vi "Example_GUI.vi"() -> ()   [LabVIEW 2016]
panel:
  in  "Device Description":string
  in  "DDS Info":T1
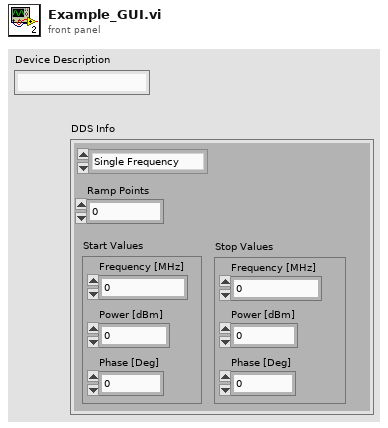
[diagram p1: front panel]
types:
  T1 = cluster{"Start Values":cluster{"Frequency [MHz]":dbl, "Power [dBm]":dbl, "Phase [Deg]":u16}, "Stop Values":cluster{"Frequency [MHz]":dbl, "Power [dBm]":dbl, "Phase [Deg]":u16}, "Ramp Points":i32, "Output Type":enum16{"Single Frequency", "Linear Ramp (dBm)"}}
  T2 = cluster{"Frequency [MHz]":dbl[], "Amplitude (0-1)":dbl[], "Phase":dbl[]}
  T3 = cluster{"Frequency 0 (MHz)":dbl[], "Frequency 1 (MHz)":dbl[], "Amplitude (0-1)":dbl[], "Phase (degrees)":dbl[], "Time (ms)":dbl[], "Sweep Direction (0 = down; 1 = up)":u16[], "Sweeps":bool, "Lock Amp":bool, "Table / Sequence":bool}
  T4 = cluster{"Frequency [MHz]":dbl, "Power [dBm]":dbl, "Phase [Deg]":u16}
  T5 = cluster{"Frequency [MHz]":dbl, "Power [dBm]":dbl, "Phase [Deg]":dbl}
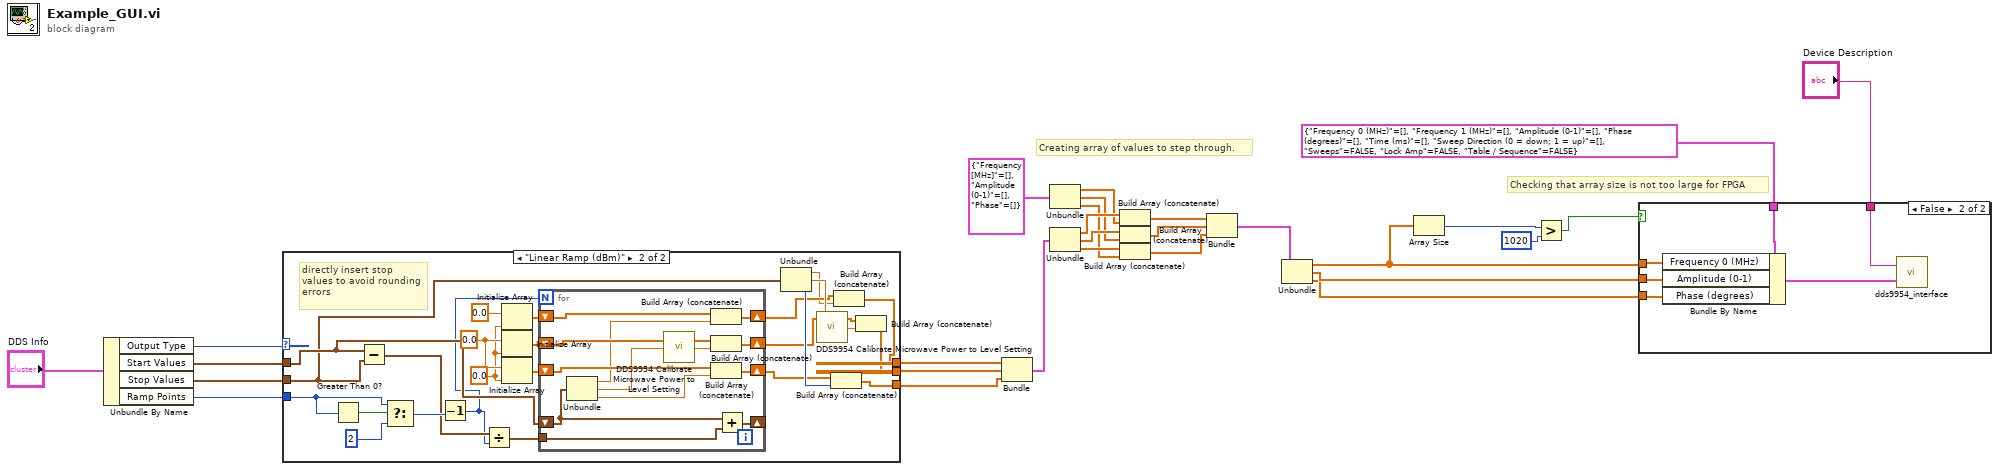
[diagram p0: block diagram]
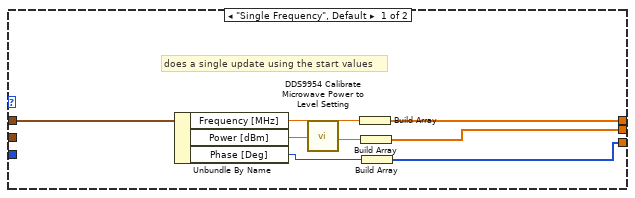
[diagram p2: hidden frame]
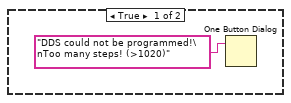
[diagram p3: hidden frame]
diagram:
  # "Checking that array size is not too large for FPGA"
  # "Creating array of values to step through."
  n1 = Unbundle By Name("DDS Info") -> ("Output Type"=w23:enum16{"Single Frequency", "Linear Ramp (dBm)"}, "Start Values"=w22:T4, "Stop Values"=w21:T4, "Ramp Points"=w20:i32)
  n2 = case shown="\"Linear Ramp (dBm)\"" w23 {
    tunnel: w22 -> [w36 w49]
    tunnel: w21 -> [_ w48]
    tunnel: w20 -> [_ w59]
    tunnel: [w33 w39] -> w19
    tunnel: [w32 w38] -> w18
    tunnel: [w31 w44] -> w17
    frame "Single Frequency", Default {
      # "does a single update using the start values"
      n3 = Unbundle By Name(w36) -> ("Frequency [MHz]"=w35:dbl, "Power [dBm]"=w29:dbl, "Phase [Deg]"=w34:u16)
      n4 = call "DDS9954 Calibrate Microwave Power to Level Setting.vi"("Desired Microwave Power [dBm]"=w29) -> ("Corresponding DDS Amplitude Fraction (0-1)"=w30:dbl)  [unwired: 4 in]
      n5 = Build Array(w35) -> (w32:dbl[])
      n6 = Build Array(w30) -> (w33:dbl[])
      n7 = Build Array(w34) -> (w31:u16[])
    }
    frame "Linear Ramp (dBm)" {
      w54 = 0.0
      w52 = 0.0 ("dimension size")
      # "directly insert stop values to avoid rounding errors"
      n8 = Greater Than 0?(x=w59) -> (x > 0?=w61:bool)
      n9 = Subtract(x=w49, y=w48) -> (x-y=w50:T4)
      n10 = Select(t=w59, s=w61, f=2) -> (s? t:f=w58:i32)
      n11 = Decrement(x=w58) -> (x-1=w37:i32)
      n12 = Divide(x=w50, y=w37) -> (x/y=w51:T5)
      n13 = Initialize Array(0.0, w52) -> (w57:dbl[])
      n14 = Initialize Array(w54, w52) -> (w56:dbl[])
      n15 = Initialize Array(w54, w52) -> (w55:dbl[])
      n16 = for {
        N: w37 -> [_]
        shift-right: [w73] -> _
        shift-left: w49 -> [w66]
        shift-right: [w71] -> w45
        shift-left: w55 -> [w72]
        tunnel: w51 -> [w74]
        shift-right: [w70] -> w41
        shift-left: w57 -> [w68]
        shift-right: [w69] -> w43
        shift-left: w56 -> [w67]
        n17 = Unbundle(w66) -> ("Frequency [MHz]"=w65:dbl, "Power [dBm]"=w64:dbl, "Phase [Deg]"=w62:dbl)
        n18 = call "DDS9954 Calibrate Microwave Power to Level Setting.vi"("Desired Microwave Power [dBm]"=w64) -> ("Corresponding DDS Amplitude Fraction (0-1)"=w63:dbl)  [unwired: 4 out]
        n19 = Build Array (concatenate)(w68, w65) -> (w70:dbl[])
        n20 = Build Array (concatenate)(w67, w63) -> (w69:dbl[])
        n21 = Build Array (concatenate)(w72, w62) -> (w71:dbl[])
        n22 = Add(x=w66, y=w74) -> (x+y=w73:T5)
      }
      n23 = Unbundle(w48) -> ("Frequency [MHz]"=w40:dbl, "Power [dBm]"=w42:dbl, "Phase [Deg]"=w46:u16)
      n24 = call "DDS9954 Calibrate Microwave Power to Level Setting.vi"("Desired Microwave Power [dBm]"=w42) -> ("Corresponding DDS Amplitude Fraction (0-1)"=w47:dbl)  [unwired: 4 out]
      n25 = Build Array (concatenate)(w45, w46) -> (w44:dbl[])
      n26 = Build Array (concatenate)(w41, w40) -> (w38:dbl[])
      n27 = Build Array (concatenate)(w43, w47) -> (w39:dbl[])
    }
  }
  n28 = Bundle(w18, w19, w17) -> (w7:cluster{dbl[], dbl[], dbl[]})  [unwired: 1 in]
  n29 = Unbundle(T2 {"Frequency [MHz]"=[], "Amplitude (0-1)"=[], "Phase"=[]} ("DDS Settings")) -> ("Frequency [MHz]"=w13:dbl[], "Amplitude (0-1)"=w12:dbl[], "Phase"=w11:dbl[])
  n30 = Unbundle(w7) -> (w16:dbl[], w15:dbl[], w14:dbl[])
  n31 = Build Array (concatenate)(w16, w13) -> (w10:dbl[])
  n32 = Build Array (concatenate)(w15, w12) -> (w9:dbl[])
  n33 = Build Array (concatenate)(w14, w11) -> (w8:dbl[])
  n34 = Bundle(w10, w9, w8) -> (w5:cluster{dbl[], dbl[], dbl[]})  [unwired: 1 out]
  n35 = Unbundle(w5) -> (w4:dbl[], w3:dbl[], w2:dbl[])
  n36 = Array Size(array=w4) -> (size(s)=w25:i32)
  n37 = Greater?(x=w25, y=1020) -> (0:w26:bool)
  n38 = case shown="False" w26 {
    tunnel: T3 {"Frequency 0 (MHz)"=[], "Frequency 1 (MHz)"=[], "Amplitude (0-1)"=[], "Phase (degrees)"=[], "Time (ms)"=[], "Sweep Direction (0 = down; 1 = up)"=[], "Sweeps"=FALSE, "Lock Amp"=FALSE, "Table / Sequence"=FALSE} -> [_ w81]
    tunnel: w4 -> [_ w80]
    tunnel: w3 -> [_ w79]
    tunnel: w2 -> [_ w78]
    tunnel: "Device Description" -> [_ w77]
    frame True {
      n39 = One Button Dialog(message="DDS could not be programmed!\nToo many steps! (>1020)") -> ()  [unwired: 1 in, 1 out]
    }
    frame False {
      n40 = Bundle By Name(cluster=w81, "Frequency 0 (MHz)"=w80, "Amplitude (0-1)"=w79, "Phase (degrees)"=w78) -> (w76:T3)
      n41 = call "dds9954_interface.vi"("DDS 9954 Interface"=w76, "Device Description"=w77) -> ()  [unwired: 8 in, 2 out]
    }
  }
